vi "OAT Digital Tacho Process (1 Tacho).vi"(0 "digital tacho info":T1={"tacho counts"=[], "counter timebase [Hz]"=1000.0, "counter task type"=enum."event counting", "counter digit (32)"=32}, 2 "reset? (F)":bool, 7 "pulse/revolution (1)":i32=1, 9 "signal duration [s]":dbl format="%0.2f", 11 "error in (no error)":errorcluster) -> (4 "speed profile":T3 {"speed [RPM]" format="%.2f"; "time [s]" format="%.2f"}, 8 "speed position info":T2, 10 "no tacho?":bool, 15 "error out":errorcluster)   [LabVIEW 2017, in "SoundVib_TachProcess.lvlib"]
doc: "Locates tachometer pulse positions in the digital tachometer signal and calculates the rotational speed of a device. Wire data to the <B>digital tacho info</B> input to determine the polymorphic instance to use or manually select the instance."
uses:
  <vilib>/addons/Sound and Vibration/Order Analysis/Tach Process/SoundVib_TachProcess.lvlib
  <vilib>/addons/Sound and Vibration/Order Analysis/Tach Process/SubVIs/speed profile.ctl
  <vilib>/addons/Sound and Vibration/Order Analysis/Misc/OAT Position Info.ctl
  <vilib>/addons/Sound and Vibration/Order Analysis/Tach Process/SubVIs/digital tach info.ctl
  <vilib>/addons/Sound and Vibration/Order Analysis/Tach Process/SubVIs/oa_Get Angular Speed (1 Tach).vi
  <vilib>/addons/Sound and Vibration/Order Analysis/Tach Process/SubVIs/oa_Process Counter Data (1 Tach).vi
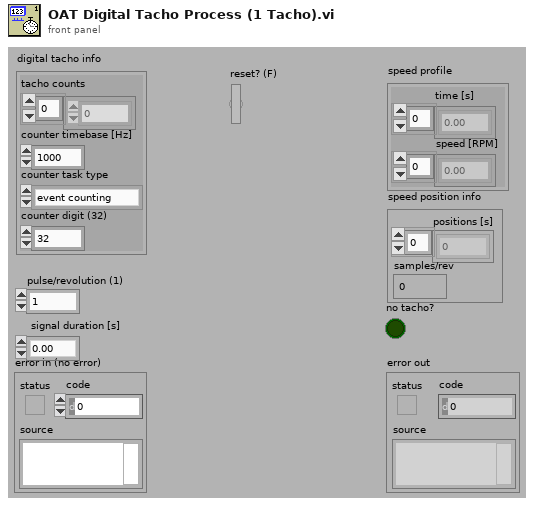
[diagram p1: front panel]
types:
  T1 = typedef "SoundVib_TachProcess.lvlib/digital tach info.ctl" = cluster{"tacho counts":i64[], "counter timebase [Hz]":dbl, "counter task type":enum16{"period measurement", "event counting"}, "counter digit (32)":i32}
  T2 = typedef "OAT Position Info.ctl" = cluster{"positions [s]":dbl[], "samples/rev":dbl}
  T3 = typedef "SoundVib_TachProcess.lvlib/speed profile.ctl" = cluster{"time [s]":dbl[], "speed [RPM]":dbl[]}
  T4 = cluster{"pulse positions [s]":dbl[], "counter timebase [Hz]":dbl, "counter task type":enum16{"period measurement", "event counting"}, "counter digit":i32}
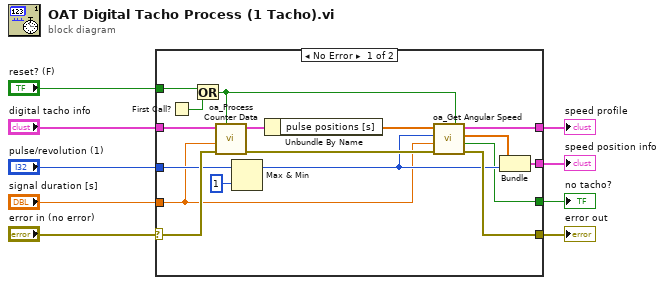
[diagram p0: block diagram]
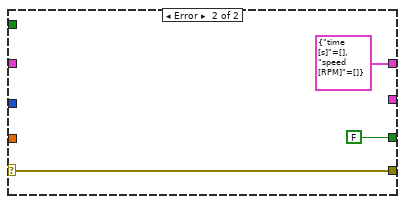
[diagram p2: hidden frame]
diagram:
  n1 = case shown="No Error" "error in (no error)" {
    selector: "error in (no error)" -> [w26 w27]
    tunnel: [w17 T3 {"time [s]"=[], "speed [RPM]"=[]} ("speed profile")] -> w9
    tunnel: [w16 w27] -> w8
    tunnel: [w10 FALSE ("No Tach? (False)")] -> w7
    tunnel: "digital tacho info" -> [w25 _]
    tunnel: "pulse/revolution (1)" -> [w22 _]
    tunnel: "reset? (F)" -> [w21 _]
    tunnel: "signal duration [s]" -> [w13 _]
    tunnel: [w24 _] -> w1
    frame No Error {
      n2 = First Call?() -> (First Call?: T/F=w20:bool)
      n3 = Or(x=w21, y=w20) -> (x .or. y?=w19:bool)
      n4 = call-poly <vilib>:"oa_Process Counter Data.vi"("reset?(True)"=w19, "error in (no error)"=w26, "vibration signal duration [s]"=w13, "digital tach info"=w25) -> ("error out (no error)"=w15:errorcluster, "digital tach info (DBL)"=w12:T4)  [unwired: 6 in]
      n5 = Max & Min(x=w22, y=1) -> (max(x,y)=w14:i32)  [unwired: 1 out]
      n6 = Unbundle By Name(w12) -> ("pulse positions [s]"=w11:dbl[])
      n7 = call-poly <vilib>:"oa_Get Angular Speed.vi"("reset? (True)"=w19, "error in (no error)"=w15, "input data duration [s]"=w13, "pulse/revolution (1)"=w14, "pulse positions [s]"=w11) -> ("error out"=w16:errorcluster, "no tacho? (F)"=w10:bool, "pulse positions [s]"=w18:dbl[], "speed profile"=w17:T3)  [unwired: 3 in]
      n8 = Bundle("pulse positions [s]"=w18, w14) -> (w24:cluster{"pulse positions [s]":dbl[], i32})  [unwired: 1 in]
    }
    frame Error {
    }
  }
  "error out" <- w8
  "speed profile" <- w9
  "speed position info" <- w1
  "no tacho?" <- w7
